vi "Serial_gets.vi"(8 "error in (no error)":errorcluster, 9 "Max Buffer Size":dbl=4000.0, 11 "Serial in":refnum<class "Serial.lvclass">) -> (0 "error out":errorcluster, 2 "String":string, 3 "Serial out":refnum<class "Serial.lvclass">)   [LabVIEW 2011, in "mbed_LVLibrary.lvlib" / "Serial.lvclass"]
doc: "Reads a string from the Serial port created on mbed until either the max buffer size is reached or a termination (\\n) is received. Note that it is best to use \"Readable\" to check for data at the Serial port before trying to read it"
uses:
  Serial.lvclass
  <vilib>/regexp/Match Regular Expression.xnode
panel:
  out "Last char":i32
  # "gets reads characters from the mbed serial port until a new line character is reached,\nthe buffer is filled or the time out occurs"
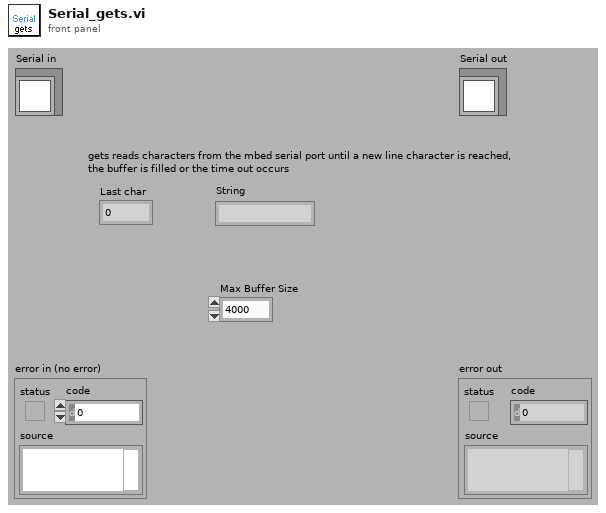
[diagram p1: front panel]
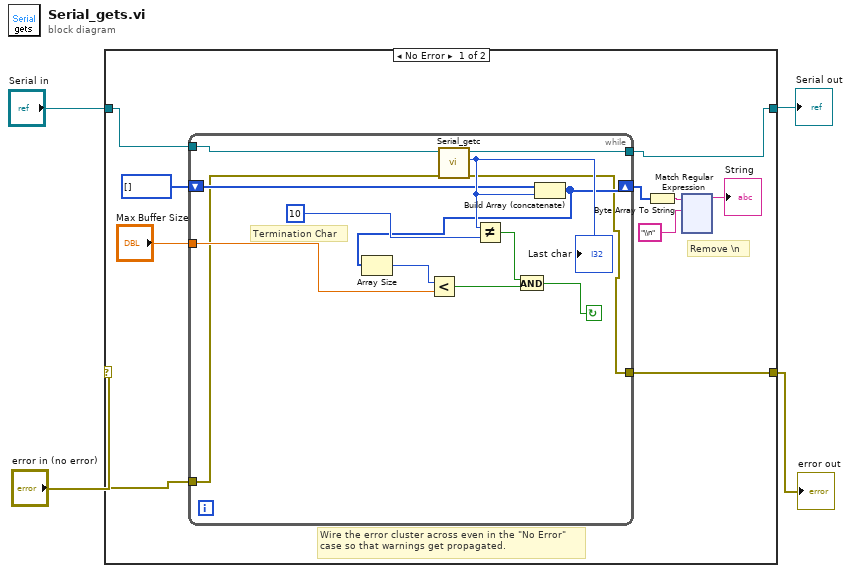
[diagram p0: block diagram]
diagram:
  n1 = case shown="No Error" "error in (no error)" {
    selector: "error in (no error)" -> [w6 w140]
    tunnel: [w5 w140] -> w3
    tunnel: [w7 w139] -> w1
    tunnel: "Serial in" -> [w8 w139]
    frame No Error {
      # "Remove \\n"
      # "Wire the error cluster across even in the \"No Error\"\ncase so that warnings get propagated."
      n2 = while {
        tunnel: "Max Buffer Size" -> [w137]
        tunnel: w8 -> [w136]
        shift-right: [w131] -> w9
        shift-left: i32[] [] -> [w130]
        tunnel: [w129] -> w7
        tunnel: w6 -> [w128]
        tunnel: [w127] -> w5
        stop <- w126 continue-if-true
        # "Termination Char"
        n3 = call "Serial_getc.vi"("error in (no error)"=w128, "Serial in"=w136) -> ("error out"=w127:errorcluster, "char"=w132:i32, "Serial out"=w129:refnum<class "Serial.lvclass">)  [unwired: 7 in]
        "Last char" <- w132
        n4 = Not Equal?(x=w132, y=10) -> (x != y?=w133:bool)
        n5 = Build Array (concatenate)(w130, w132) -> (w131:i32[])
        n6 = Array Size(array=w131) -> (size(s)=w138:i32)
        n7 = Less?(x=w138, y=w137) -> (x < y?=w135:bool)
        n8 = And(x=w133, y=w135) -> (x .and. y?=w126:bool)
      }
      n9 = Byte Array To String(unsigned byte array=w9) -> (string=w12:string)
      n10 = xnode "Match Regular Expression"("input string"=w12, "regular expression"="\\n") -> ("before match"=→"String":string)  [unwired: 4 in, 4 out]
    }
    frame Error {
    }
  }
  "error out" <- w3
  "Serial out" <- w1
